vi "Configure Channel (RTD Scale).vi"(0 "VISA resource name":refnum<visa-resource-name>, 1 "Scaling":T1={"Floating point position (2)"=2, "Lower Scaling (0)"=0.0, "Upper Scaling (100.00)"=100.0, "Unit Character (\"\")"=""} {"Upper Scaling (100.00)" format="%_6g"; "Lower Scaling (0)" format="%_6g"; "Floating point position (2)" min=0 max=5 step=1}, 5 "Channel (0001)":string="0001", 7 "Enable Channel (True)":bool=TRUE, 9 "Type and Span":T2={"RTD Type (0 : Pt100)"=0, "Enable Span (False)"=FALSE, "Lower Span (-200.0)"=-200.0, "Upper Span (850.0)"=850.0, "Bias (0)"=0.0} {"Bias (0)" format="%_6g"; "Upper Span (850.0)" min=-99999.0 max=99999.0 step=0.1 format="%.2f"; "Lower Span (-200.0)" min=-99999.0 max=99999.0 step=0.1 format="%.2f"; "RTD Type (0 : Pt100)" items=["Pt100", "Pt100-H", "JPt100", "JPt100-H", "Cu10GE", "Cu10LN", "Cu10WEED", "Cu10BAILEY", "Cu10a392", "Cu10a393", "Cu25", "Cu53", "Cu100", "J263B", "Ni100SAMA", "Ni100DIN", "Ni120", "Pt25", "Pt50", "Pt200WEED", "Cu10G", "Cu50G", "Cu100G", "Pt46G", "Pt100G"]}, 11 "error in (no error)":errorcluster) -> (4 "VISA resource name out":refnum<visa-resource-name>, 6 "channel":string, 15 "error out":errorcluster)   [LabVIEW 2020, in "Yokogawa GX Series.lvlib"]
doc: "Sets the input range as Resistance Temperature Detector (RTD).\n\nCommand: SRangeAI"
uses:
  <instrlib>/Yokogawa GX Series/Yokogawa GX Series.lvlib
  <instrlib>/Yokogawa GX Series/Private/RTD Range.vi
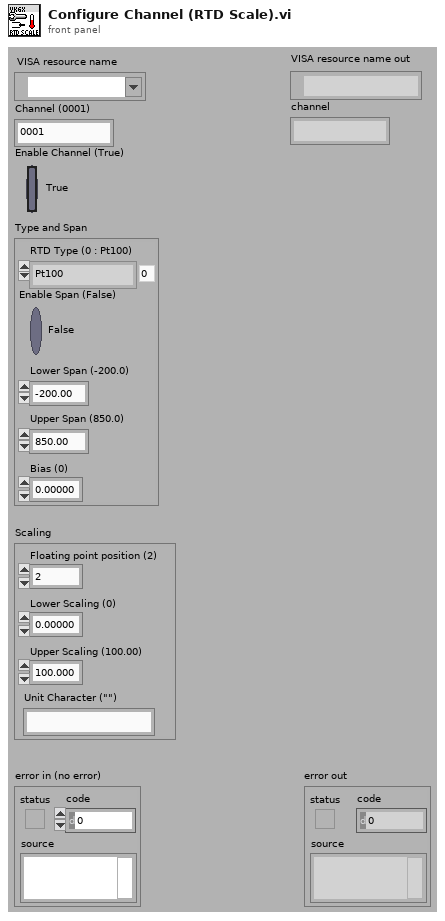
[diagram p1: front panel]
types:
  T1 = cluster{"Floating point position (2)":i32, "Lower Scaling (0)":dbl, "Upper Scaling (100.00)":dbl, "Unit Character (\"\")":string}
  T2 = cluster{"RTD Type (0 : Pt100)":i32, "Enable Span (False)":bool, "Lower Span (-200.0)":dbl, "Upper Span (850.0)":dbl, "Bias (0)":dbl}
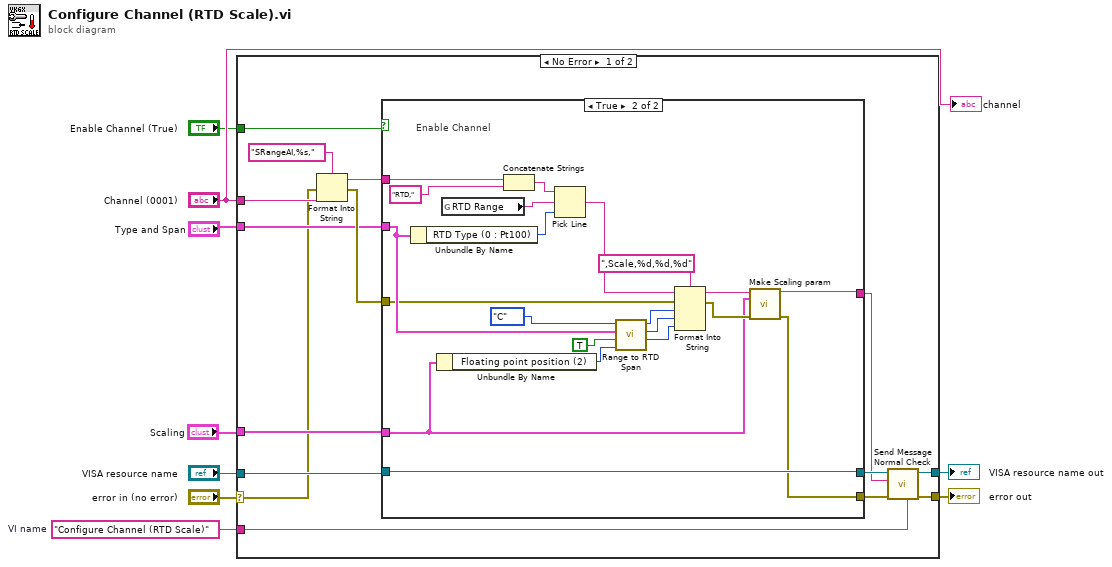
[diagram p0: block diagram]
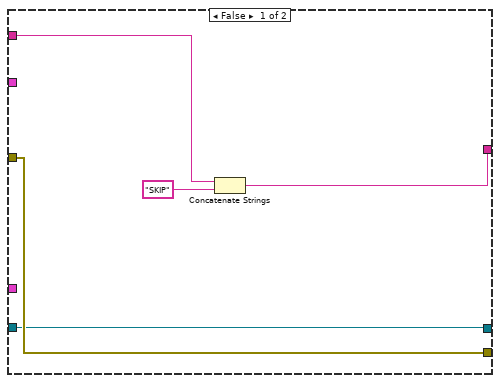
[diagram p2: hidden frame]
diagram:
  w2 = "Configure Channel (RTD Scale)"  # VI name
  n1 = case shown="No Error" "error in (no error)" {
    selector: "error in (no error)" -> [w10 w51]
    tunnel: "VISA resource name" -> [w21 w52]
    tunnel: "Type and Span" -> [w20 _]
    tunnel: [w17 w52] -> w7
    tunnel: [w16 w51] -> w6
    tunnel: "Scaling" -> [w14 _]
    tunnel: "Channel (0001)" -> [w13 _]
    tunnel: "Enable Channel (True)" -> [w12 _]
    tunnel: w2 -> [w11 _]
    frame No Error {
      n2 = Format Into String(format string="SRangeAI,%s,", error in=w10, w13) -> (resulting string=w22:string, error out=w23:errorcluster)  [unwired: 1 in]
      n3 = case shown="True" w12 {
        tunnel: w23 -> [w28 w41]
        tunnel: w22 -> [w29 w49]
        tunnel: [w28 w32] -> w18
        tunnel: w21 -> [w27 w42]
        tunnel: [w27 w42] -> w19
        tunnel: w20 -> [_ w47]
        tunnel: [w26 w33] -> w15
        tunnel: w14 -> [_ w34]
        frame False {
          n4 = Concatenate Strings(w29, "SKIP") -> (w26:string)
        }
        frame True {
          # "Enable Channel"
          n5 = Unbundle By Name(w47) -> ("RTD Type (0 : Pt100)"=w46:i32)
          n6 = Unbundle By Name(w34) -> ("Floating point position (2)"=w38:i32)
          n7 = global read "RTD Range.vi" "RTD Range"() -> (w30:string)
          n8 = Concatenate Strings(w49, "RTD,") -> (w48:string)
          n9 = Pick Line(string ("")=w48, multi-line string=w30, line index=w46) -> (output string=w45:string)
          n10 = call <instrlib>:"Range to RTD Span.vi"("Floating Point Position (2)"=w38, "Scaling? (False)"=TRUE, "Type and Span"=w47, "Temp. unit (0: C)"=enum16{"C", "F"}."C") -> ("Bias"=w43:i32, "Upper span"=w37:i32, "Lower Span"=w44:i32)  [unwired: 5 in]
          n11 = Format Into String(format string=",Scale,%d,%d,%d", initial string=w45, error in=w41, w44, w37, w43) -> (resulting string=w36:string, error out=w35:errorcluster)
          n12 = call <instrlib>:"Make Scaling param.vi"("String (\"\")"=w36, "Scaling"=w34, "error in (no error)"=w35) -> ("String After"=w33:string, "error out"=w32:errorcluster)  [unwired: 11 in]
        }
      }
      n13 = call <instrlib>:"Send Message Normal Check.vi"("Source (\"\")"=w11, "error in (no error)"=w18, "Send Message (\"\")"=w15, "VISA resource name"=w19) -> ("error out"=w16:errorcluster, "VISA resource name out"=w17:refnum<visa-resource-name>)  [unwired: 2 in, 4 out]
    }
    frame Error {
    }
  }
  "error out" <- w6
  "VISA resource name out" <- w7
  "channel" <- "Channel (0001)"
